vi "Autonomous Independent.vi"() -> ()   [LabVIEW 2011]
doc: "This VI is called when autonomous begins, and will automatically be terminated when autonomous ends. You can carry out timed or sensor driven robot movement independently without needing to return to the caller."
uses:
  Controls/Robot Orientation.ctl
  Autonomous/Auto Drive Emulation.vi
  Globals/Autonomous Tipping.vi
  Globals/Autonomous Joystick Emulation.vi
  Globals/DriveSystemMode.vi
  Globals/Max Robot Speed.vi
  Globals/Image Height.vi
panel:
  in  "Stop Auto":bool
  out "Command":dbl
  out "Traveled":dbl
  out "Done":bool
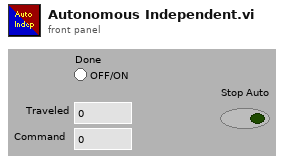
[diagram p1: front panel]
types:
  T1 = typedef "Robot Orientation.ctl" = enum16{"Landscape", "Portrait"}
  T2 = typedef "Drive System Mode.ctl" = enum16{"Normal", "Crab", "Shoot"}
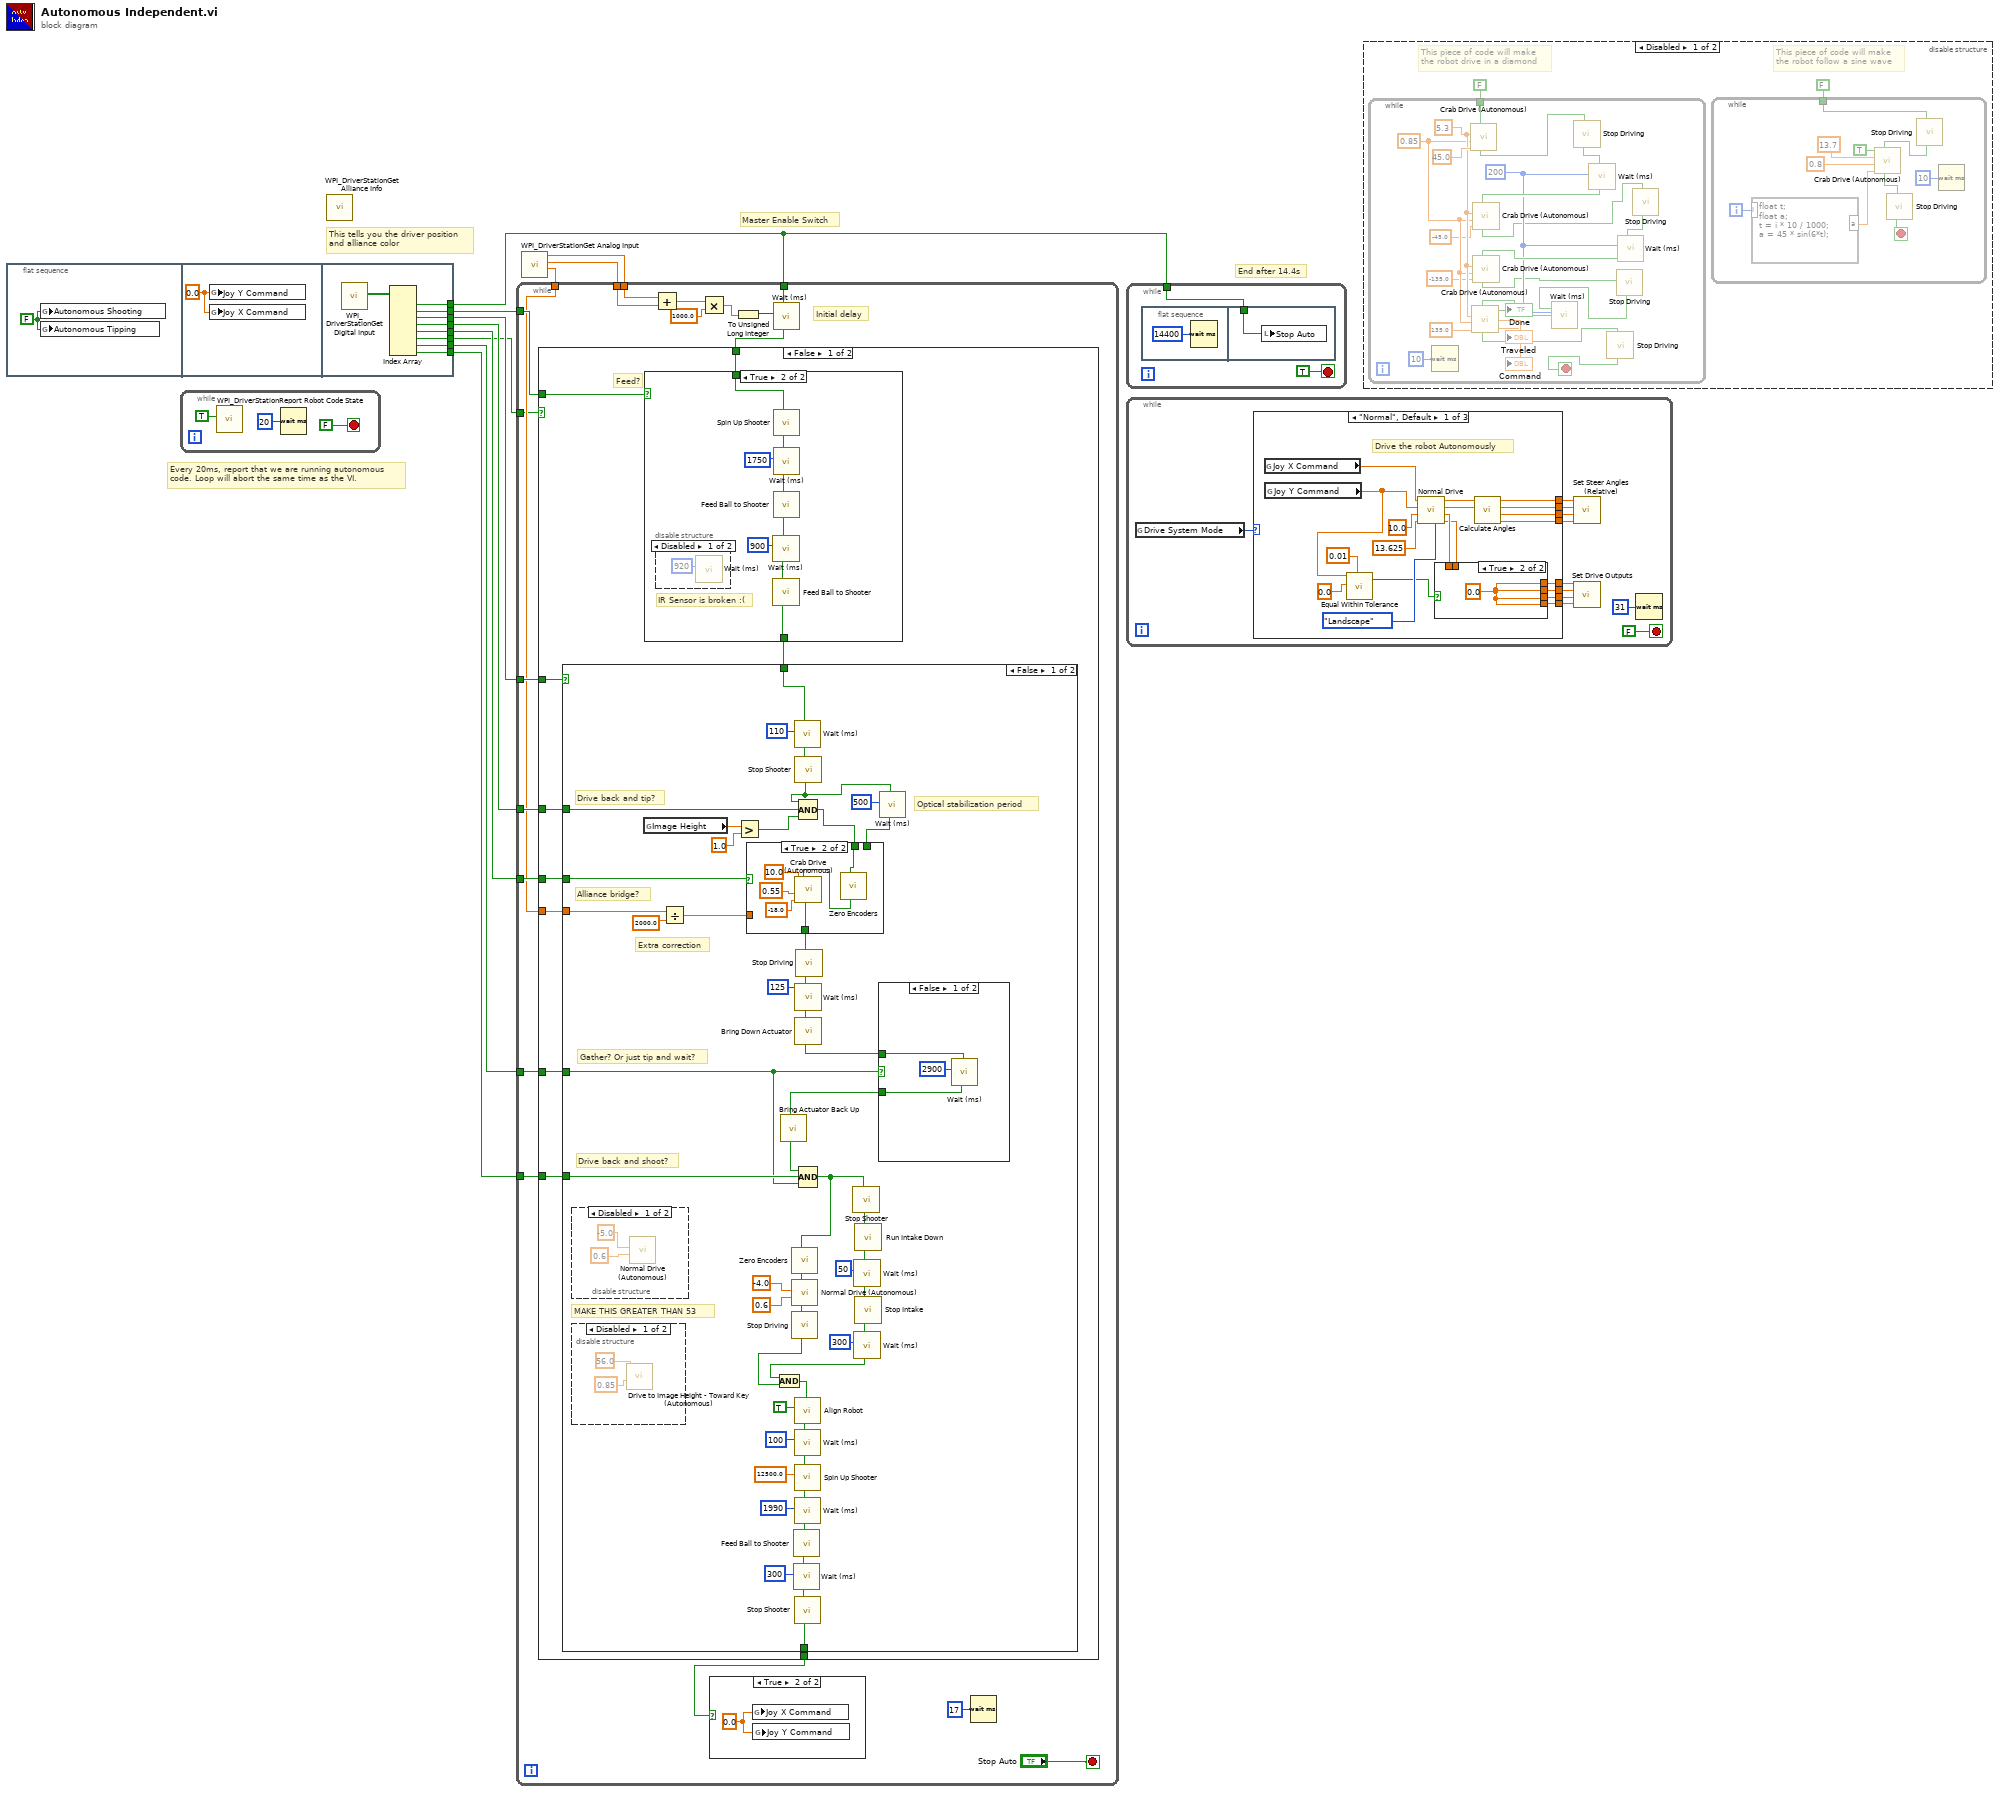
[diagram p0: block diagram]
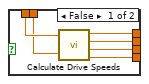
[diagram p3: hidden frame]
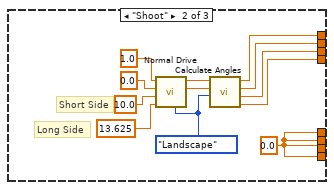
[diagram p4: hidden frame]
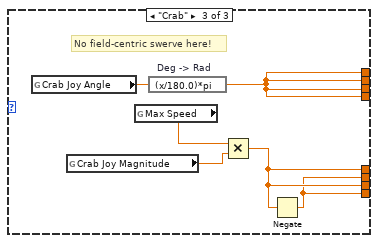
[diagram p5: hidden frame]
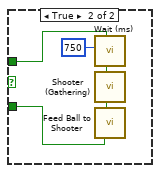
[diagram p8: hidden frame]
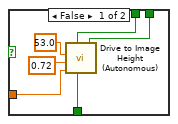
[diagram p9: hidden frame]
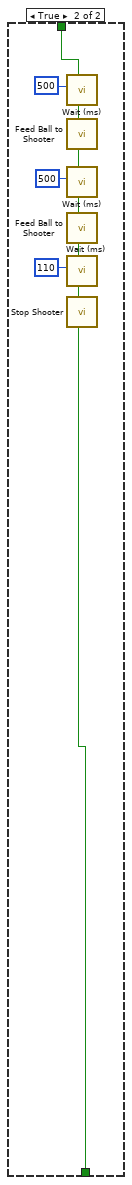
[diagram p12: hidden frame]
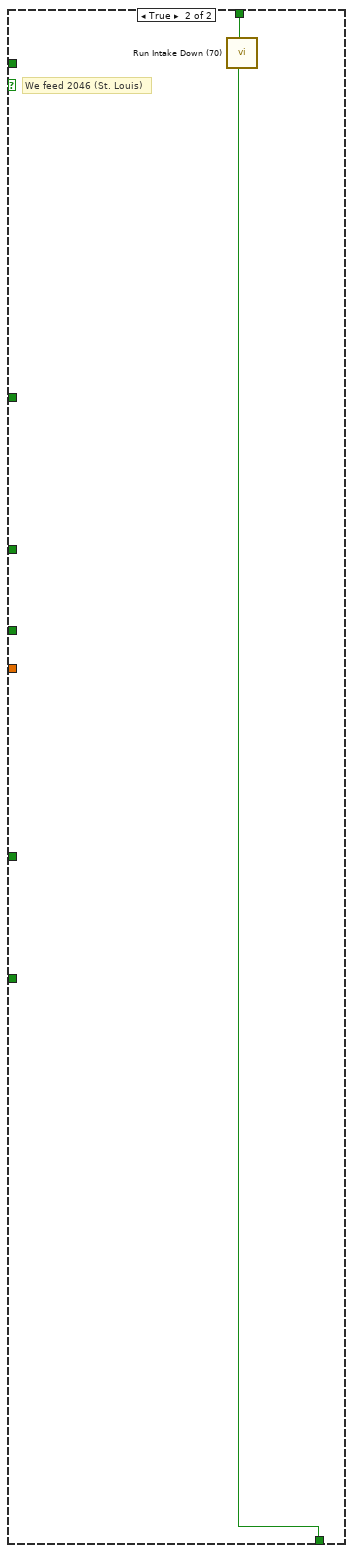
[diagram p13: hidden frame]
diagram:
  # "End after 14.4s"
  # "Master Enable Switch"
  # "Every 20ms, report that we are running autonomous\ncode. Loop will abort the same time as the VI."
  # "This tells you the driver position\nand alliance color"
  n1 = flat-sequence {
    tunnel: [w21] -> w1
    tunnel: [w20] -> w11
    tunnel: [w19] -> w10
    tunnel: [w18] -> w9
    tunnel: [w17] -> w6
    tunnel: [w16] -> w5
    tunnel: [w15] -> w4
    tunnel: [w14] -> w2
    frame #0 {
      w12 = FALSE ("Autonomous Tipping")
      n2 = global write "Auto Drive Emulation.vi" "Autonomous Shooting"(w12) -> ()
      n3 = global write "Autonomous Tipping.vi" "Autonomous Tipping"(w12) -> ()
    }
    frame #1 {
      w13 = 0.0 ("Joy Y Command")
      n4 = global write "Autonomous Joystick Emulation.vi" "Joy Y Command"(w13) -> ()
      n5 = global write "Autonomous Joystick Emulation.vi" "Joy X Command"(w13) -> ()
    }
    frame #2 {
      n6 = call <vilib>:"WPI_DriverStationGet Digital Input.vi"() -> ("Driver Station Digital Input (1-8)"=w22:bool[])  [unwired: 11 out]
      n7 = Index Array(array=w22) -> (element #1=w21:bool, element #2=w15:bool, element #3=w20:bool, element #4=w19:bool, element #5=w18:bool, element #6=w14:bool, element #7=w16:bool, element #8=w17:bool)  [unwired: 8 in]
    }
  }
  n8 = while {
    stop <- FALSE stop-if-true
    n9 = call <vilib>:"WPI_DriverStationReport Robot Code State.vi"("Autonomous"=TRUE) -> ()  [unwired: 10 in, 1 out]
    n10 = Wait (ms)(milliseconds to wait=u32 20) -> ()  [unwired: 1 out]
  }
  n11 = call <vilib>:"WPI_DriverStationGet Alliance Info.vi"() -> ()  [unwired: 12 out]
  n12 = call <vilib>:"WPI_DriverStationGet Analog Input.vi"() -> ("Analog 3 (V)"=w3:dbl, "Analog 2 (V)"=w7:dbl, "Analog 1 (V)"=w8:dbl)  [unwired: 9 out]
  n13 = while {
    tunnel: w1 -> [w42]
    tunnel: w11 -> [w40]
    tunnel: w10 -> [w39]
    tunnel: w9 -> [w38]
    tunnel: w8 -> [w35]
    tunnel: w7 -> [w34]
    tunnel: w6 -> [w31]
    tunnel: w5 -> [w30]
    tunnel: w4 -> [w29]
    tunnel: w3 -> [w28]
    tunnel: w2 -> [w27]
    stop <- "Stop Auto" stop-if-true
    # "Initial delay"
    n14 = Add(x=w35, y=w34) -> (x+y=w37:dbl)
    n15 = Multiply(x=w37, y=1000.0 ("x+y")) -> (x*y=w32:dbl)
    n16 = To Unsigned Long Integer(number=w32) -> (unsigned 32bit integer=w33:u32)
    n17 = call "Wait (ms).vi"("Execute"=w42, "milliseconds to wait"=w33) -> ("Done Executing"=w43:bool)  [unwired: 6 in]
    n18 = case shown="False" w27 {
      tunnel: w43 -> [w54 w150]
      tunnel: [w52 w149] -> w41
      tunnel: w40 -> [w51 _]
      tunnel: w39 -> [w50 _]
      tunnel: w38 -> [w49 _]
      tunnel: w31 -> [w48 _]
      tunnel: w30 -> [w47 _]
      tunnel: w29 -> [w46 _]
      tunnel: w28 -> [w45 _]
      frame False {
        # "Feed?"
        n19 = case shown="True" w46 {
          tunnel: w54 -> [w55 w63]
          tunnel: [w55 w56] -> w53
          frame False {
          }
          frame True {
            # "IR Sensor is broken :("
            n20 = disable-structure shown="Disabled" {
              frame Disabled {
                n21 = call "Wait (ms).vi"("milliseconds to wait"=u32 920) -> ()  [unwired: 7 in, 1 out]
              }
              frame Enabled {
              }
            }
            n22 = call "Spin Up Shooter.vi"("Execute"=w63) -> ("Done Executing"=w61:bool)  [unwired: 7 in]
            n23 = call "Wait (ms).vi"("Execute"=w61, "milliseconds to wait"=u32 1750) -> ("Done Executing"=w59:bool)  [unwired: 6 in]
            n24 = call "Feed Ball to Shooter.vi"("Execute"=w59) -> ("Done Executing"=w58:bool)  [unwired: 7 in]
            n25 = call "Wait (ms).vi"("Execute"=w58, "milliseconds to wait"=u32 900) -> ("Done Executing"=w57:bool)  [unwired: 6 in]
            n26 = call "Feed Ball to Shooter.vi"("Execute"=w57) -> ("Done Executing"=w56:bool)  [unwired: 7 in]
          }
        }
        n27 = case shown="False" w51 {
          tunnel: w53 -> [w81 w140]
          tunnel: [w82 w139] -> w52
          tunnel: w50 -> [w80 _]
          tunnel: w49 -> [w79 _]
          tunnel: w48 -> [w78 _]
          tunnel: w47 -> [w70 _]
          tunnel: w45 -> [w67 _]
          frame False {
            # "Extra correction"
            # "Alliance bridge?"
            # "Drive back and tip?"
            # "Gather? Or just tip and wait?"
            # "MAKE THIS GREATER THAN 53"
            # "Drive back and shoot?"
            # "Optical stabilization period"
            n28 = disable-structure shown="Disabled" {
              frame Disabled {
                n29 = call "Normal Drive (Autonomous).vi"("Distance (Feet)"=-5.0, "Percent Speed"=0.6) -> ()  [unwired: 3 in, 4 out]
              }
              frame Enabled {
              }
            }
            n30 = disable-structure shown="Disabled" {
              frame Disabled {
                n31 = call "Drive to Image Height - Toward Key (Autonomous).vi"("Image Height (Pixels)"=56.0, "Percent Velocity"=0.85) -> ()  [unwired: 6 in, 1 out]
              }
              frame Enabled {
              }
            }
            n32 = global read "Image Height.vi" "Image Height"() -> (w85:dbl)
            n33 = Divide(x=w67, y=2000.0) -> (x/y=w66:dbl)
            n34 = Greater?(x=w85, y=1.0) -> (0:w84:bool)
            n35 = call "Wait (ms).vi"("Execute"=w81, "milliseconds to wait"=u32 110) -> ("Done Executing"=w109:bool)  [unwired: 6 in]
            n36 = call "Stop Shooter.vi"("Execute"=w109) -> ("Done Executing"=w90:bool)  [unwired: 7 in]
            n37 = Compound Arithmetic op=AND(w90, w80, w84) -> (w108:bool)
            n38 = call "Wait (ms).vi"("Execute"=w90, "milliseconds to wait"=u32 500) -> ("Done Executing"=w91:bool)  [unwired: 6 in]
            n39 = case shown="True" w79 {
              tunnel: [w128 w134] -> w111
              tunnel: w108 -> [w125 w130]
              tunnel: w91 -> [w124 _]
              tunnel: w66 -> [w123 _]
              frame False {
                n40 = call "Drive to Image Height (Autonomous).vi"("Execute"=w125, "Image Height (Pixels)"=53.0, "Percent Velocity"=0.72, "Extra Correction"=w123, "Camera Stabilized?"=w124) -> ("Done Executing"=w128:bool)  [unwired: 3 in]
              }
              frame True {
                n41 = call "Zero Encoders.vi"("Execute"=w130) -> ("Done Executing"=w129:bool)  [unwired: 7 in]
                n42 = call "Crab Drive (Autonomous).vi"("Execute"=w129, "Distance (Feet)"=10.0, "Percent Speed"=0.55, "Angle (Degrees)"=-18.0) -> ("Done Executing"=w134:bool)  [unwired: 1 in, 3 out]
              }
            }
            n43 = call "Stop Driving.vi"("Execute"=w111) -> ("Done Executing"=w113:bool)  [unwired: 7 in]
            n44 = call "Wait (ms).vi"("Execute"=w113, "milliseconds to wait"=u32 125) -> ("Done Executing"=w112:bool)  [unwired: 6 in]
            n45 = call "Bring Down Actuator.vi"("Execute"=w112) -> ("Done Executing"=w73:bool)  [unwired: 7 in]
            n46 = case shown="False" w70 {
              tunnel: w73 -> [w116 w119]
              tunnel: [w115 w118] -> w72
              frame False {
                n47 = call "Wait (ms).vi"("Execute"=w116, "milliseconds to wait"=u32 2900) -> ("Done Executing"=w115:bool)  [unwired: 6 in]
              }
              frame True {
                n48 = call "Wait (ms).vi"("Execute"=w119, "milliseconds to wait"=u32 750) -> ("Done Executing"=w120:bool)  [unwired: 6 in]
                n49 = call "Shooter (Gathering).vi"("Execute"=w120) -> ("Done Executing"=w122:bool)  [unwired: 7 in]
                n50 = call "Feed Ball to Shooter.vi"("Execute"=w122) -> ("Done Executing"=w118:bool)  [unwired: 7 in]
              }
            }
            n51 = call "Bring Actuator Back Up.vi"("Execute"=w72) -> ("Done Executing"=w83:bool)  [unwired: 7 in]
            n52 = Compound Arithmetic op=AND(w83, w78, w70) -> (w75:bool)
            n53 = call "Zero Encoders.vi"("Execute"=w75) -> ("Done Executing"=w76:bool)  [unwired: 7 in]
            n54 = call "Normal Drive (Autonomous).vi"("Execute"=w76, "Distance (Feet)"=-4.0, "Percent Speed"=0.6) -> ("Done Executing"=w69:bool)  [unwired: 2 in, 3 out]
            n55 = call "Stop Driving.vi"("Execute"=w69) -> ("Done Executing"=w68:bool)  [unwired: 7 in]
            n56 = call "Stop Shooter.vi"("Execute"=w75) -> ("Done Executing"=w93:bool)  [unwired: 7 in]
            n57 = call "Run Intake Down.vi"("Execute"=w93) -> ("Done Executing"=w105:bool)  [unwired: 7 in]
            n58 = call "Wait (ms).vi"("Execute"=w105, "milliseconds to wait"=u32 50) -> ("Done Executing"=w104:bool)  [unwired: 6 in]
            n59 = call "Stop Intake.vi"("Execute"=w104) -> ("Done Executing"=w103:bool)  [unwired: 7 in]
            n60 = call "Wait (ms).vi"("Execute"=w103, "milliseconds to wait"=u32 300) -> ("Done Executing"=w71:bool)  [unwired: 6 in]
            n61 = And(x=w71, y=w68) -> (x .and. y?=w97:bool)
            n62 = call "Align Robot.vi"("Execute"=w97, "Autonomous Shooting"=TRUE) -> ("Done Executing"=w98:bool)  [unwired: 6 in]
            n63 = call "Wait (ms).vi"("Execute"=w98, "milliseconds to wait"=u32 100) -> ("Done Executing"=w96:bool)  [unwired: 6 in]
            n64 = call "Spin Up Shooter.vi"("Execute"=w96, "Manual Speed"=12500.0) -> ("Done Executing"=w88:bool)  [unwired: 6 in]
            n65 = call "Wait (ms).vi"("Execute"=w88, "milliseconds to wait"=u32 1990) -> ("Done Executing"=w94:bool)  [unwired: 6 in]
            n66 = call "Feed Ball to Shooter.vi"("Execute"=w94) -> ("Done Executing"=w102:bool)  [unwired: 7 in]
            n67 = call "Wait (ms).vi"("Execute"=w102, "milliseconds to wait"=u32 300) -> ("Done Executing"=w100:bool)  [unwired: 6 in]
            n68 = call "Stop Shooter.vi"("Execute"=w100) -> ("Done Executing"=w82:bool)  [unwired: 7 in]
          }
          frame True {
            n69 = call "Wait (ms).vi"("Execute"=w140, "milliseconds to wait"=u32 500) -> ("Done Executing"=w145:bool)  [unwired: 6 in]
            n70 = call "Feed Ball to Shooter.vi"("Execute"=w145) -> ("Done Executing"=w141:bool)  [unwired: 7 in]
            n71 = call "Wait (ms).vi"("Execute"=w141, "milliseconds to wait"=u32 500) -> ("Done Executing"=w142:bool)  [unwired: 6 in]
            n72 = call "Feed Ball to Shooter.vi"("Execute"=w142) -> ("Done Executing"=w148:bool)  [unwired: 7 in]
            n73 = call "Wait (ms).vi"("Execute"=w148, "milliseconds to wait"=u32 110) -> ("Done Executing"=w147:bool)  [unwired: 6 in]
            n74 = call "Stop Shooter.vi"("Execute"=w147) -> ("Done Executing"=w139:bool)  [unwired: 7 in]
          }
        }
      }
      frame True {
        # "We feed 2046 (St. Louis)"
        n75 = call "Run Intake Down (70).vi"("Execute"=w150) -> ("Done Executing"=w149:bool)  [unwired: 7 in]
      }
    }
    n76 = case shown="True" w41 {
      frame False {
      }
      frame True {
        w151 = 0.0 ("Joy X Command")
        n77 = global write "Autonomous Joystick Emulation.vi" "Joy X Command"(w151) -> ()
        n78 = global write "Autonomous Joystick Emulation.vi" "Joy Y Command"(w151) -> ()
      }
    }
    n79 = Wait (ms)(milliseconds to wait=u32 17) -> ()  [unwired: 1 out]
  }
  n80 = while {
    tunnel: w1 -> [w152]
    stop <- TRUE stop-if-true
    n81 = flat-sequence {
      tunnel: w152 -> [w155]
      frame #0 {
        n82 = Wait (ms)(milliseconds to wait=u32 14400) -> ()  [unwired: 1 out]
      }
      frame #1 {
        n83 = local write "Stop Auto"(w155) -> ()
      }
    }
  }
  n84 = while {
    stop <- FALSE stop-if-true
    n85 = global read "DriveSystemMode.vi" "Drive System Mode"() -> (w164:T2)
    n86 = case shown="\"Normal\", Default" w164 {
      tunnel: [w174 w198 w210] -> w163
      tunnel: [w173 w198 w209] -> w162
      tunnel: [w172 w198 w210] -> w161
      tunnel: [w171 w198 w209] -> w160
      tunnel: [w170 w197 w208] -> w159
      tunnel: [w169 w196 w208] -> w158
      tunnel: [w168 w195 w208] -> w157
      tunnel: [w167 w194 w208] -> w156
      frame "Normal", Default {
        # "Drive the robot Autonomously"
        n87 = global read "Autonomous Joystick Emulation.vi" "Joy X Command"() -> (w175:dbl)
        n88 = global read "Autonomous Joystick Emulation.vi" "Joy Y Command"() -> (w176:dbl)
        n89 = call "Equal Within Tolerance.vi"("Number In"=w176, "Comparison Value"=0.0, "Tolerance"=0.01) -> ("Equality"=w177:bool)  [unwired: 16 in]
        n90 = call "Normal Drive.vi"("Joy X"=w175, "Joy Y"=w176, "Short Radius (Inches)"=10.0 ("Vertical Radius (Inches)"), "Long Radius (Inches)"=13.625 ("Lateral Radius (Inches)"), "Robot Orientation"=Robot_Orientation."Landscape") -> ("Front Left Angle Out"=w186:dbl, "Front Right Angle Out"=w185:dbl, "Left Speed Out"=w184:dbl, "Right Speed Out"=w183:dbl)  [unwired: 1 in]
        n91 = case shown="True" w177 {
          tunnel: [w192 w193] -> w174
          tunnel: [w191 w193] -> w173
          tunnel: [w190 w193] -> w172
          tunnel: [w189 w193] -> w171
          tunnel: w184 -> [w188 _]
          tunnel: w183 -> [w187 _]
          frame False {
            n92 = call "Calculate Drive Speeds.vi"("Left Speed In"=w188, "Right Speed In"=w187) -> ("Front Left Speed"=w192:dbl, "Front Right Speed"=w191:dbl, "Rear Left Speed"=w190:dbl, "Rear Right Speed"=w189:dbl)  [unwired: 2 in]
          }
          frame True {
            w193 = 0.0 ("Front Left Speed")
          }
        }
        n93 = call "Calculate Angles.vi"("Right Angle In"=w185, "Left Angle In"=w186) -> ("Rear Right Steer Out"=w167:dbl, "Rear Left Pot Out"=w168:dbl, "Front Right Pot Out"=w169:dbl, "Front Left Pot Out"=w170:dbl)  [unwired: 2 in]
      }
      frame "Shoot" {
        w198 = 0.0 ("Front Left Speed")
        w199 = Robot_Orientation."Landscape" ("Robot Orientation")
        # "Long Side"
        # "Short Side"
        n94 = call "Normal Drive.vi"("Joy X"=1.0, "Joy Y"=0.0, "Short Radius (Inches)"=10.0 ("Vertical Radius (Inches)"), "Long Radius (Inches)"=13.625 ("Lateral Radius (Inches)"), "Robot Orientation"=w199) -> ("Front Left Angle Out"=w201:dbl, "Front Right Angle Out"=w200:dbl)  [unwired: 1 in, 2 out]
        n95 = call "Calculate Angles.vi"("Robot Orientation"=w199, "Right Angle In"=w200, "Left Angle In"=w201) -> ("Rear Right Steer Out"=w194:dbl, "Rear Left Pot Out"=w195:dbl, "Front Right Pot Out"=w196:dbl, "Front Left Pot Out"=w197:dbl)  [unwired: 1 in]
      }
      frame "Crab" {
        # "No field-centric swerve here!"
        n96 = global read "Autonomous Joystick Emulation.vi" "Crab Joy Angle"() -> (w207:dbl)
        n97 = global read "Autonomous Joystick Emulation.vi" "Crab Joy Magnitude"() -> (w206:dbl)
        n98 = global read "Max Robot Speed.vi" "Max Speed"() -> (w211:dbl)
        n99 = expression code="(x/180.0)*pi" "Deg -> Rad"(w207) -> (w208:dbl)
        n100 = Multiply(x=w211, y=w206) -> (x*y=w210:dbl)
        n101 = Negate(x=w210) -> (-x=w209:dbl)
      }
    }
    n102 = call "Set Steer Angles (Relative).vi"("Rear Right"=w156, "Rear Left"=w157, "Front Right"=w158, "Front Left"=w159) -> ()  [unwired: 8 in]
    n103 = call "Set Drive Outputs.vi"("Front Left"=w163, "Front Right"=w162, "Rear Left"=w161, "Rear Right"=w160) -> ()  [unwired: 24 in]
    n104 = Wait (ms)(milliseconds to wait=u32 31) -> ()  [unwired: 1 out]
  }
  n105 = disable-structure shown="Disabled" {
    frame Disabled {
      # "This piece of code will make\nthe robot follow a sine wave"
      # "This piece of code will make\nthe robot drive in a diamond"
      n106 = while {
        tunnel: FALSE -> [w235]
        stop <- w227 stop-if-true
        w241 = u32 200 ("milliseconds to wait")
        w239 = 0.85 ("Percent Speed")
        w240 = 5.3 ("Distance (Feet)")
        n107 = Wait (ms)(milliseconds to wait=u32 10) -> ()  [unwired: 1 out]
        n108 = call "Crab Drive (Autonomous).vi"("Execute"=w235, "Distance (Feet)"=w240, "Percent Speed"=w239, "Angle (Degrees)"=45.0) -> ("Done Executing"=w234:bool)  [unwired: 1 in, 3 out]
        n109 = call "Stop Driving.vi"("Execute"=w234) -> ("Done Executing"=w233:bool)  [unwired: 7 in]
        n110 = call "Wait (ms).vi"("Execute"=w233, "milliseconds to wait"=w241) -> ("Done Executing"=w244:bool)  [unwired: 6 in]
        n111 = call "Crab Drive (Autonomous).vi"("Execute"=w244, "Distance (Feet)"=w240, "Percent Speed"=w239, "Angle (Degrees)"=-45.0) -> ("Done Executing"=w232:bool)  [unwired: 1 in, 3 out]
        n112 = call "Stop Driving.vi"("Execute"=w232) -> ("Done Executing"=w231:bool)  [unwired: 7 in]
        n113 = call "Wait (ms).vi"("Execute"=w231, "milliseconds to wait"=w241) -> ("Done Executing"=w243:bool)  [unwired: 6 in]
        n114 = call "Crab Drive (Autonomous).vi"("Execute"=w243, "Distance (Feet)"=w240, "Percent Speed"=w239, "Angle (Degrees)"=-135.0) -> ("Done Executing"=w230:bool)  [unwired: 1 in, 3 out]
        n115 = call "Stop Driving.vi"("Execute"=w230) -> ("Done Executing"=w229:bool)  [unwired: 7 in]
        n116 = call "Wait (ms).vi"("Execute"=w229, "milliseconds to wait"=w241) -> ("Done Executing"=w242:bool)  [unwired: 6 in]
        n117 = call "Crab Drive (Autonomous).vi"("Execute"=w242, "Distance (Feet)"=w240, "Percent Speed"=w239, "Angle (Degrees)"=135.0) -> ("Done Executing"=w228:bool, "Done"=→"Done":bool, "Traveled"=→"Traveled":dbl, "Command"=→"Command":dbl)  [unwired: 1 in]
        n118 = call "Stop Driving.vi"("Execute"=w228) -> ("Done Executing"=w227:bool)  [unwired: 7 in]
      }
      n119 = while {
        tunnel: FALSE -> [w215]
        i -> [w220]
        stop <- w217 stop-if-true
        n120 = formula code="float t;\nfloat a;\nt = i * 10 / 1000;\na = 45 * sin(6*t);"("i"=w220) -> ("a"=w219:dbl)
        n121 = call "Stop Driving.vi"("Execute"=w215) -> ("Done Executing"=w214:bool)  [unwired: 7 in]
        n122 = call "Crab Drive (Autonomous).vi"("Ignore Turning?"=TRUE, "Execute"=w214, "Distance (Feet)"=13.7, "Percent Speed"=0.8, "Angle (Degrees)"=w219) -> ("Done Executing"=w218:bool)  [unwired: 3 out]
        n123 = call "Stop Driving.vi"("Execute"=w218) -> ("Done Executing"=w217:bool)  [unwired: 7 in]
        n124 = Wait (ms)(milliseconds to wait=u32 10) -> ()  [unwired: 1 out]
      }
    }
    frame Enabled {
    }
  }
